vi "P-Latch Ascent.vi"(10 "Input":bool, 11 "Enum":enum16{"Start", "Run", "End"}(ring)) -> (3 "Latched":bool)   [LabVIEW 2012]
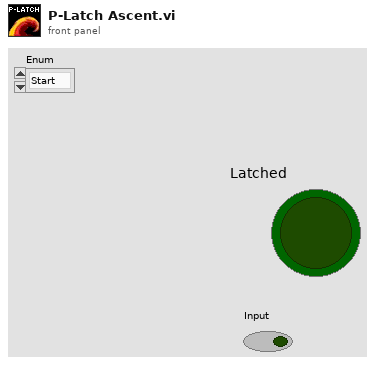
[diagram p1: front panel]
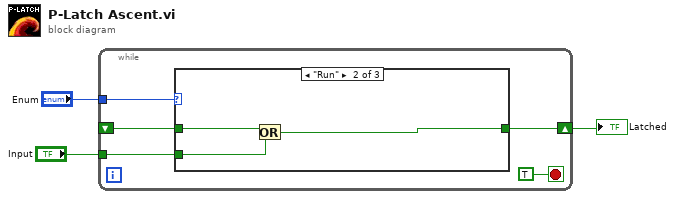
[diagram p0: block diagram]
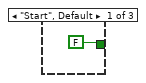
[diagram p2: hidden frame]
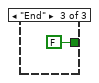
[diagram p3: hidden frame]
diagram:
  n1 = while {
    tunnel: "Input" -> [w7]
    shift-right: [w6] -> w2
    shift-left: _ -> [w5]
    tunnel: "Enum" -> [w4]
    stop <- TRUE stop-if-true
    n2 = case shown="\"Run\"" w4 {
      tunnel: w7 -> [_ w12 _]
      tunnel: [FALSE w11 FALSE] -> w6
      tunnel: w5 -> [_ w10 _]
      frame "Start", Default {
      }
      frame "Run" {
        n3 = Or(x=w10, y=w12) -> (x .or. y?=w11:bool)
      }
      frame "End" {
      }
    }
  }
  "Latched" <- w2
